vi "Test3v3.vi"() -> ()   [LabVIEW 2013]
panel:
  out "Lengths":string[](array[string])
  out "Leen 5 cout":i32
  out "appended array":string[](array[string])
  out "index":i32
  out "*(type *) &x":string
  out "size(s)":i32
  out "hex integer string":string[](array[string])
  in  "error in":errorcluster
  out "error out":errorcluster
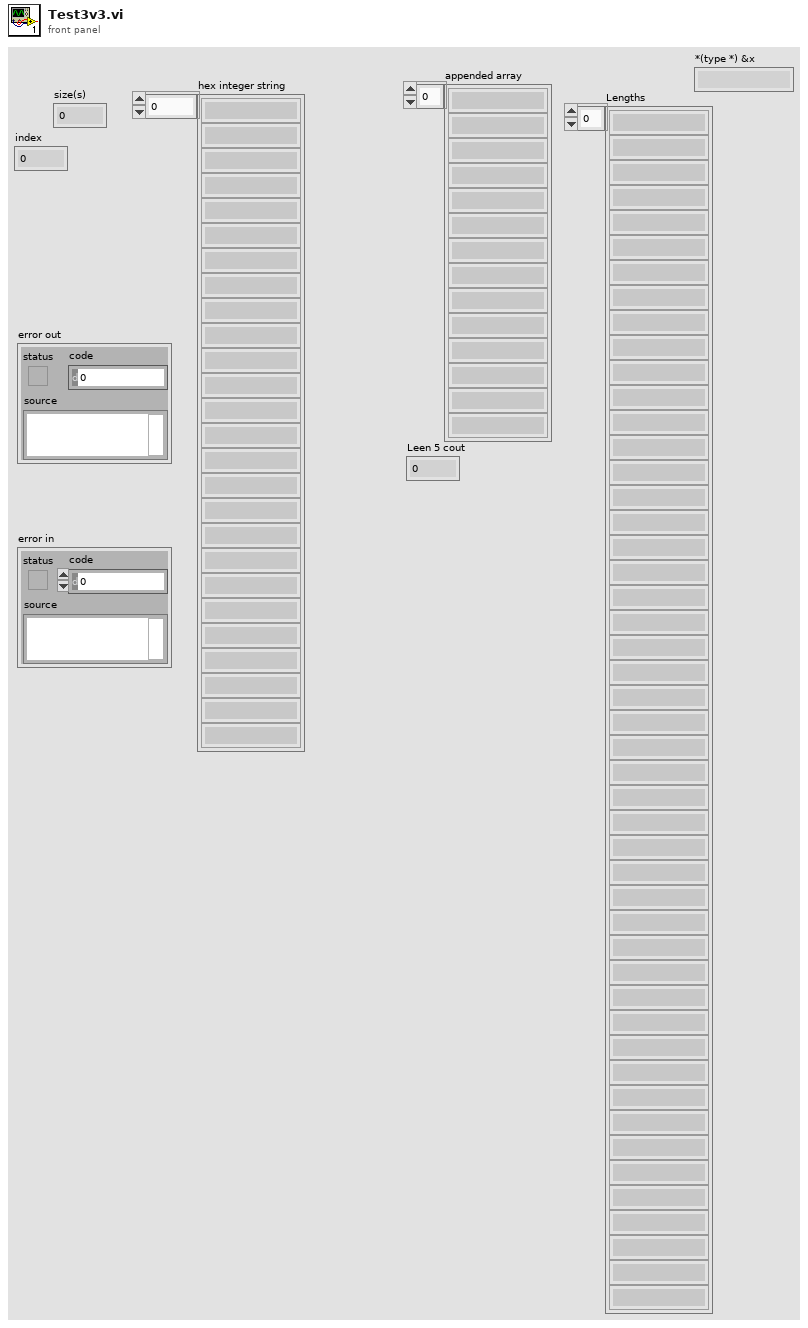
[diagram p1: front panel]
types:
  T1 = enum16{"big-endian, network order", "native, host order", "little-endian"}
  T2 = enum16{"open", "replace", "create", "open or create", "replace or create", "replace or create with confirmation"}
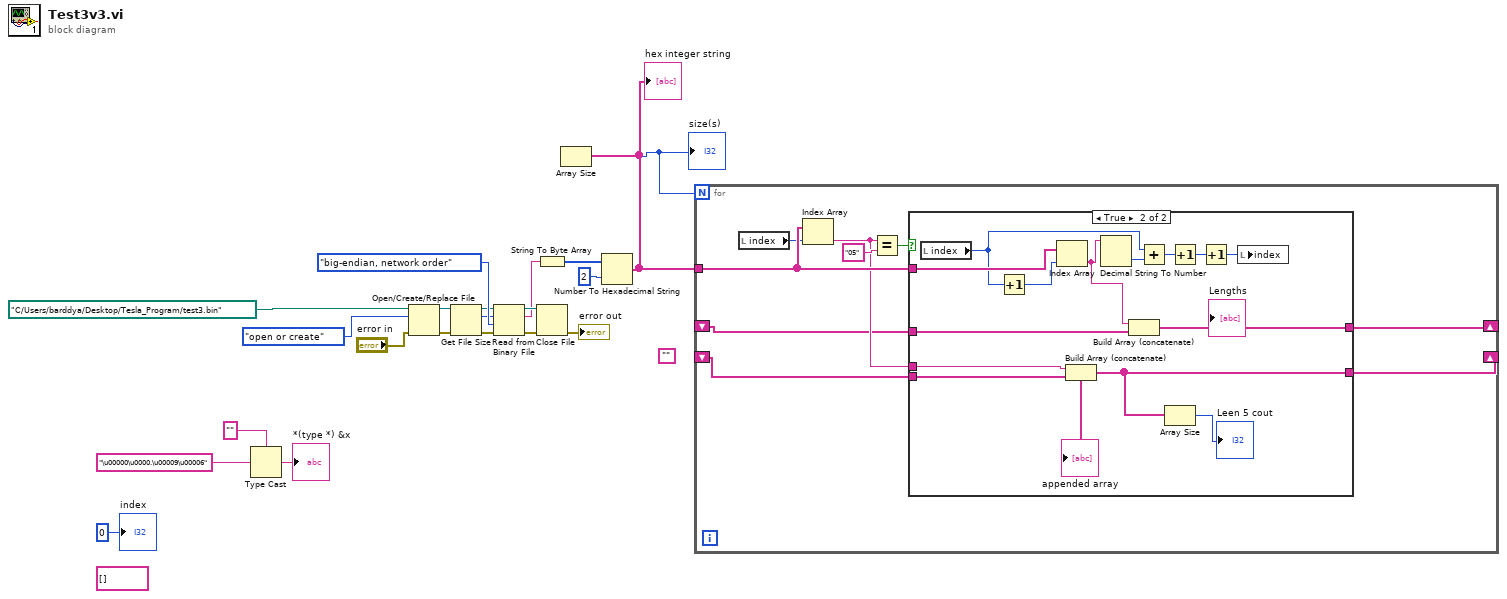
[diagram p0: block diagram]
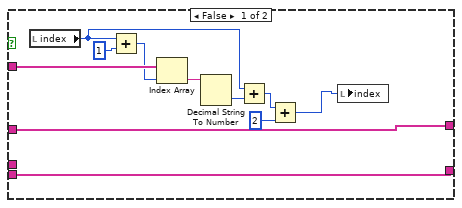
[diagram p2: hidden frame]
diagram:
  (unwired) ""
  (unwired) string[] [] ("subarray")
  n1 = Type Cast(type="", x="\u00000\u0000.\u00009\u00006") -> (*(type *) &x=→"*(type *) &x":string)
  n2 = Open/Create/Replace File(file path (use dialog)=path "C:/Users/barddya/Desktop/Tesla_Program/test3.bin", error in="error in", operation (0:open)=T2."open or create") -> (refnum out=w14:refnum<file>, error out=w12:errorcluster)  [unwired: 3 in, 1 out]
  n3 = Get File Size(file=w14, error in=w12) -> (refnum out=w13:refnum<file>, size (in bytes)=w10:i64, 0:w11:errorcluster)
  n4 = Read from Binary File(8:w11, 9:T1."big-endian, network order" ("byte order (0:big-endian, network order)"), 10:w10, 11:w13) -> (0:w17:errorcluster, 2:w9:string, 3:w15:refnum<file>)  [unwired: 2 in, 1 out]
  n5 = String To Byte Array(string=w9) -> (unsigned byte array=w8:u8[])
  n6 = Close File(refnum=w15, error in=w17) -> (error out=→"error out":errorcluster)  [unwired: 1 out]
  n7 = Number To Hexadecimal String(1:2, 2:w8) -> (0:w3:string[])
  "hex integer string" <- w3
  n8 = Array Size(array=w3) -> (size(s)=w1:i32)
  "size(s)" <- w1
  n9 = for {
    N: w1 -> [_]
    tunnel: w3 -> [w28]
    shift-right: [w25] -> _
    shift-left: _ -> [w24]
    shift-right: [w23] -> _
    shift-left: _ -> [w22]
    n10 = local read "index"() -> (w27:i32)
    n11 = Index Array(array=w28, index=w27) -> (element=w26:string)
    n12 = Equal?(x=w26, y="05") -> (x = y?=w29:bool)
    n13 = case shown="True" w29 {
      tunnel: w28 -> [w39 w55]
      tunnel: w26 -> [_ w50]
      tunnel: [w32 w46] -> w25
      tunnel: w24 -> [w32 w49]
      tunnel: [w31 w44] -> w23
      tunnel: w22 -> [w31 w47]
      frame False {
        n14 = local read "index"() -> (w36:i32)
        n15 = Add(x=w36, y=1) -> (x+y=w37:i32)
        n16 = Index Array(array=w39, index=w37) -> (element=w41:string)
        n17 = Decimal String To Number(string=w41) -> (number=w40:i32)  [unwired: 2 in, 1 out]
        n18 = Add(x=w36, y=w40) -> (x+y=w35:i32)
        n19 = Add(x=w35, y=2) -> (x+y=w33:i32)
        n20 = local write "index"(w33) -> ()
      }
      frame True {
        n21 = local read "index"() -> (w53:i32)
        n22 = Increment(x=w53) -> (x+1=w54:i32)
        n23 = Index Array(array=w55, index=w54) -> (element=w42:string)
        n24 = Build Array (concatenate)(w50, w49) -> (w46:string[])
        "appended array" <- w46
        n25 = Decimal String To Number(string=w42) -> (number=w48:i32)  [unwired: 2 in, 1 out]
        n26 = Build Array (concatenate)(w42, w47) -> (w44:string[])
        "Lengths" <- w44
        n27 = Add(x=w53, y=w48) -> (x+y=w43:i32)
        n28 = Array Size(array=w46) -> (size(s)=→"Leen 5 cout":i32)
        n29 = Increment(x=w43) -> (x+1=w52:i32)
        n30 = Increment(x=w52) -> (x+1=w51:i32)
        n31 = local write "index"(w51) -> ()
      }
    }
  }
  "index" <- 0
